vi "Get Script Name.vi"() -> (3 "Script Name":string)   [LabVIEW 2014]
uses:
  <vilib>/Rock Robotics/WPI/DriverStation/WPI_DriverStationRobotMode2.ctl
  <vilib>/Rock Robotics/Network Tables/SD Read Boolean.vi
  Begin/Global Variables.vi
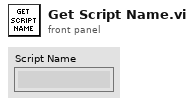
[diagram p1: front panel]
types:
  T1 = typedef "WPI_DriverStationRobotMode2.ctl" = enum16{"Autonomous Disabled", "Autonomous Enabled", "Teleop Disabled", "Teleop Enabled", "Disconnected", "Finish", "Test Disabled", "Test Enabled", "Emergency Stopped"}
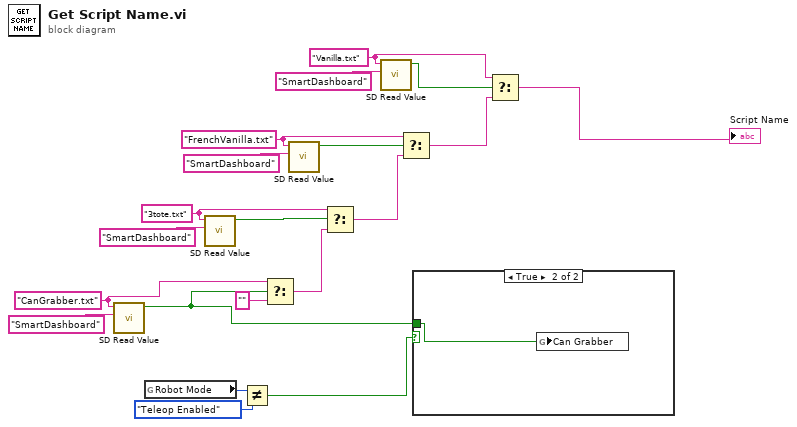
[diagram p0: block diagram]
diagram:
  w6 = "CanGrabber.txt" ("Name")
  w10 = "3tote.txt" ("Name")
  w13 = "FrenchVanilla.txt" ("Name")
  w15 = "Vanilla.txt" ("Name")
  n1 = call-poly <vilib>:"SD Read Value.vi"("Table Prefix"="SmartDashboard", "Name"=w6) -> ("Boolean"=w1:bool)  [unwired: 7 in, 2 out]
  n2 = global read "Global Variables.vi" "Robot Mode"() -> (w4:T1)
  n3 = call-poly <vilib>:"SD Read Value.vi"("Table Prefix"="SmartDashboard", "Name"=w10) -> ("Boolean"=w11:bool)  [unwired: 7 in, 2 out]
  n4 = Not Equal?(x=w4, y=WPI_DriverStationRobotMode2."Teleop Enabled") -> (x != y?=w2:bool)
  n5 = Select(t=w6, s=w1, f="") -> (s? t:f=w7:string)
  n6 = call-poly <vilib>:"SD Read Value.vi"("Table Prefix"="SmartDashboard", "Name"=w13) -> ("Boolean"=w12:bool)  [unwired: 7 in, 2 out]
  n7 = Select(t=w10, s=w11, f=w7) -> (s? t:f=w9:string)
  n8 = call-poly <vilib>:"SD Read Value.vi"("Table Prefix"="SmartDashboard", "Name"=w15) -> ("Boolean"=w16:bool)  [unwired: 7 in, 2 out]
  n9 = Select(t=w13, s=w12, f=w9) -> (s? t:f=w14:string)
  n10 = case shown="True" w2 {
    tunnel: w1 -> [_ w21]
    frame False {
    }
    frame True {
      n11 = global write "Global Variables.vi" "Can Grabber"(w21) -> ()
    }
  }
  n12 = Select(t=w15, s=w16, f=w14) -> (s? t:f=→"Script Name":string)
